vi "GetAttributeViBoolean_SA-Marker_Source.vi"(8 "error in (no error)":errorcluster {"code" format="%.0x"}, 9 "AttributeID":u32(ring)=1150703 items=["SA_MARKER_CONTINUOUS_PEAK_SEARCH_ENABLED"=1150703, "SA_MARKER_COUPLE_ENABLED"=1150689, "SA_MARKER_ENABLED"=1150691, "SA_MARKER_FREQUENCYCOUNTER_GATE_TIME_AUTO_ENABLED"=1150684, "SA_MARKER_FREQUENCYCOUNTER_RESOLUTION_AUTO_ENABLED"=1150685, "SA_MARKER_FUNCTION_BAND_SPAN_AUTO_ENABLED"=1150704, "SA_MARKER_LINES_ENABLED"=1150696, "SA_MARKER_MEASUREATMARKER_COUPLE_ENABLED"=1150753, "SA_MARKER_MEASUREATMARKER_PRESELECTOR_CENTERING_ENABLED"=1150755, "SA_MARKER_NDBPOINTS_ENABLED"=1150686, "SA_MARKER_PEAK_EXCURSION_ENABLED"=1150706, "SA_MARKER_PEAK_TABLE_ENABLED"=1150697, "SA_MARKER_SIGNAL_TRACK_ENABLED"=1150718, "SA_MARKER_TABLE_ENABLED"=1150700, "SA_MARKER_THRESHOLD_ENABLED"=1150705, "SA_MARKER_TRACE_AUTO_ENABLED"=1150701, "SA_MARKER_X_AXIS_SCALE_AUTO_ENABLED"=1150699, "SA_SOURCE_FREQUENCY_OFFSET_ENABLED"=1150798, "SA_SOURCE_FREQUENCY_SWEEP_REVERSE_ENABLED"=1150796, "SA_SOURCE_LEVEL_AMPLITUDE_STEP_AUTO_ENABLED"=1150792, "SA_SOURCE_LEVEL_POWER_SWEEP_ENABLED"=1150789, "SA_SOURCE_RF_OUTPUT_ENABLED"=1150784], 11 "instrument handle":refnum<k15>) -> (0 "error out":errorcluster {"code" format="%.0x"}, 2 "AttributeValue":bool, 3 "instrument handle out":refnum<k15>)   [LabVIEW 2009, in "Keysight XSAn.lvlib"]
doc: "Gets a Boolean attribute from the instrument driver.\nThe following Attributes are supported:\n\nSA_MARKER_CONTINUOUS_PEAK_SEARCH_ENABLED\nSA_MARKER_COUPLE_ENABLED\nSA_MARKER_ENABLED\nSA_MARKER_FREQUENCYCOUNTER_GATE_TIME_AUTO_ENABLED\nSA_MARKER_FREQUENCYCOUNTER_RESOLUTION_AUTO_ENABLED\nSA_MARKER_FUNCTION_BAND_SPAN_AUTO_ENABLED\nSA_MARKER_LINES_ENABLED\nSA_MARKER_MEASUREATMARKER_COUPLE_ENABLED\nSA_MARKER_MEASUREATMARKER_PRESELECTOR_CENTERING_ENABLED\nSA_MARKER_NDBPOINTS_ENABLED\nSA_MARKER_PEAK_EXCURSION_ENABLED\nSA_MARKER_PEAK_TABLE_ENABLED\nSA_MARKER_SIGNAL_TRACK_ENABLED\nSA_MARKER_TABLE_ENABLED\nSA_MARKER_THRESHOLD_ENABLED\nSA_MARKER_TRACE_AUTO_ENABLED\nSA_MARKER_X_AXIS_SCALE_AUTO_ENABLED\nSA_SOURCE_FREQUENCY_OFFSET_ENABLED\nSA_SOURCE_FREQUENCY_SWEEP_REVERSE_ENABLED\nSA_SOURCE_LEVEL_AMPLITUDE_STEP_AUTO_ENABLED\nSA_SOURCE_LEVEL_POWER_SWEEP_ENABLED\nSA_SOURCE_RF_OUTPUT_ENABLED"
uses:
  <instrlib>/Keysight XSAn/Keysight XSAn.lvlib
  AgXSAn.dll
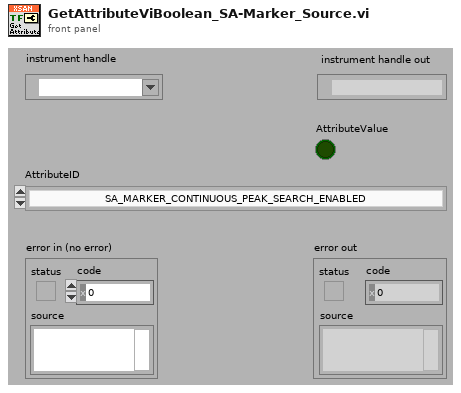
[diagram p1: front panel]
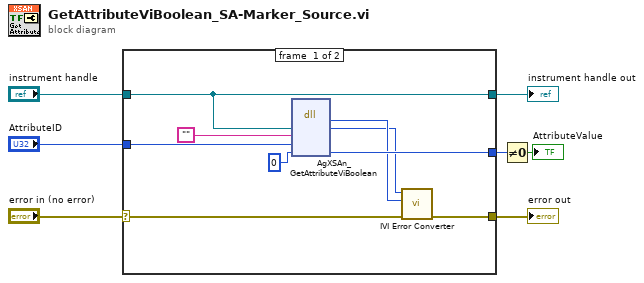
[diagram p0: block diagram]
diagram:
  n1 = case shown="No Error" "error in (no error)" {
    selector: "error in (no error)" -> [w16 w18]
    tunnel: [w15 w18] -> w7
    tunnel: "instrument handle" -> [w11 w17]
    tunnel: "AttributeID" -> [w14 _]
    tunnel: [w12 _] -> w2
    tunnel: [w11 w17] -> w1
    frame #0 {
      n2 = dll-call lib="AgXSAn**.dll" fn="AgXSAn_GetAttributeViBoolean"("Vi"=w11, "RepCapIdentifier"="", "AttributeID"=w14, "AttributeValue"=i16 0) -> ("return type"=w10:i32, "Vi"=w9:u32, "AttributeValue"=w12:i16)  [unwired: 5 in, 2 out]
      n3 = call <instrlib>:"IVI Error Converter.vi"("error in (no error)"=w16, "IVI error code (0)"=w10, "instrument handle"=w9) -> ("error out"=w15:errorcluster)  [unwired: 7 in, 1 out]
    }
    frame #1 {
    }
  }
  "error out" <- w7
  "instrument handle out" <- w1
  n4 = Not Equal To 0?(x=w2) -> (x != 0?=→"AttributeValue":bool)
